vi "REF_EDITOR_records_click_discard.vi"(10 "CellPosition":T2, 11 "event_structure_shift_register_in":T1={"REF_EDIT_clicked_row"=-1, "REF_EDIT_selected_row"=-1, "SQL_EDIT_clicked_row"=-1, "SQL_EDIT_selected_row"=-1, "ARCH_EDIT_selected_row"=-1, "ARCH_EDIT_clicked_row"=-1, "USER_EDIT_selected_row"=-1, "USER_EDIT_clicked_row"=-1, "REPORT_GEAR_toggle_all_results"=FALSE}) -> (2 "Discard?":bool, 3 "event_structure_shift_register_out":T1={"REF_EDIT_clicked_row"=-1, "REF_EDIT_selected_row"=-1, "SQL_EDIT_clicked_row"=-1, "SQL_EDIT_selected_row"=-1, "ARCH_EDIT_selected_row"=-1, "ARCH_EDIT_clicked_row"=-1, "USER_EDIT_selected_row"=-1, "USER_EDIT_clicked_row"=-1, "REPORT_GEAR_toggle_all_results"=FALSE})   [LabVIEW 2019]
uses:
  CLIENT_event_structure_shift_register.ctl
  <vilib>/Utility/miscctls.llb/LVRowAndColumnTypeDef.ctl
  FGV/REF_EDITOR_records_display/FGV_REF_EDITOR_records_display.ctl
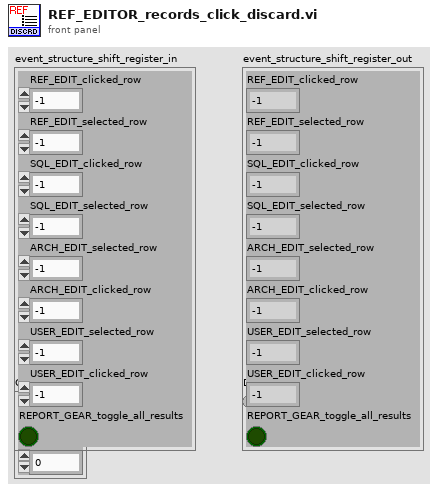
[diagram p1: front panel]
types:
  T1 = typedef "CLIENT_event_structure_shift_register.ctl" = cluster{"REF_EDIT_clicked_row":i32, "REF_EDIT_selected_row":i32, "SQL_EDIT_clicked_row":i32, "SQL_EDIT_selected_row":i32, "ARCH_EDIT_selected_row":i32, "ARCH_EDIT_clicked_row":i32, "USER_EDIT_selected_row":i32, "USER_EDIT_clicked_row":i32, "REPORT_GEAR_toggle_all_results":bool}
  T2 = typedef "LVRowAndColumnTypeDef.ctl" = cluster{"Row":i32, "Column":i32}
  T3 = typedef "FGV_REF_EDITOR_records_display.ctl" = enum16{"initialize", "set_reference_tables_names", "set_station_number", "set_type_filter", "set_headers", "set_records", "get_ref_table_name", "get_ref_hist_table_name", "get_station_number", "get_type_filter", "get_headers", "get_uneditable_columns", "get_all_info", "record_added?", "record_inserted?", "record_edited?", "record_updated?", "record_deleted?", "discard_changes"}
  T4 = typedef "REF_EDITOR_all_info.ctl" = cluster{"station_number":string, "type_filter":string, "reference_table":string, "reference_history":string, "headers":string[], "uneditable_columns":string[], "uneditable_columns":i32[], "editable_columns":i32[], "values_in_database":string[][], "size":cluster{"columns":i32, "SQL_rows":i32, "disp_rows":i32}, "REF_record_states":T5[]}
  T5 = typedef "SQL_record_states.ctl" = enum16{"Equal", "Added", "Edited", "Deleted"}
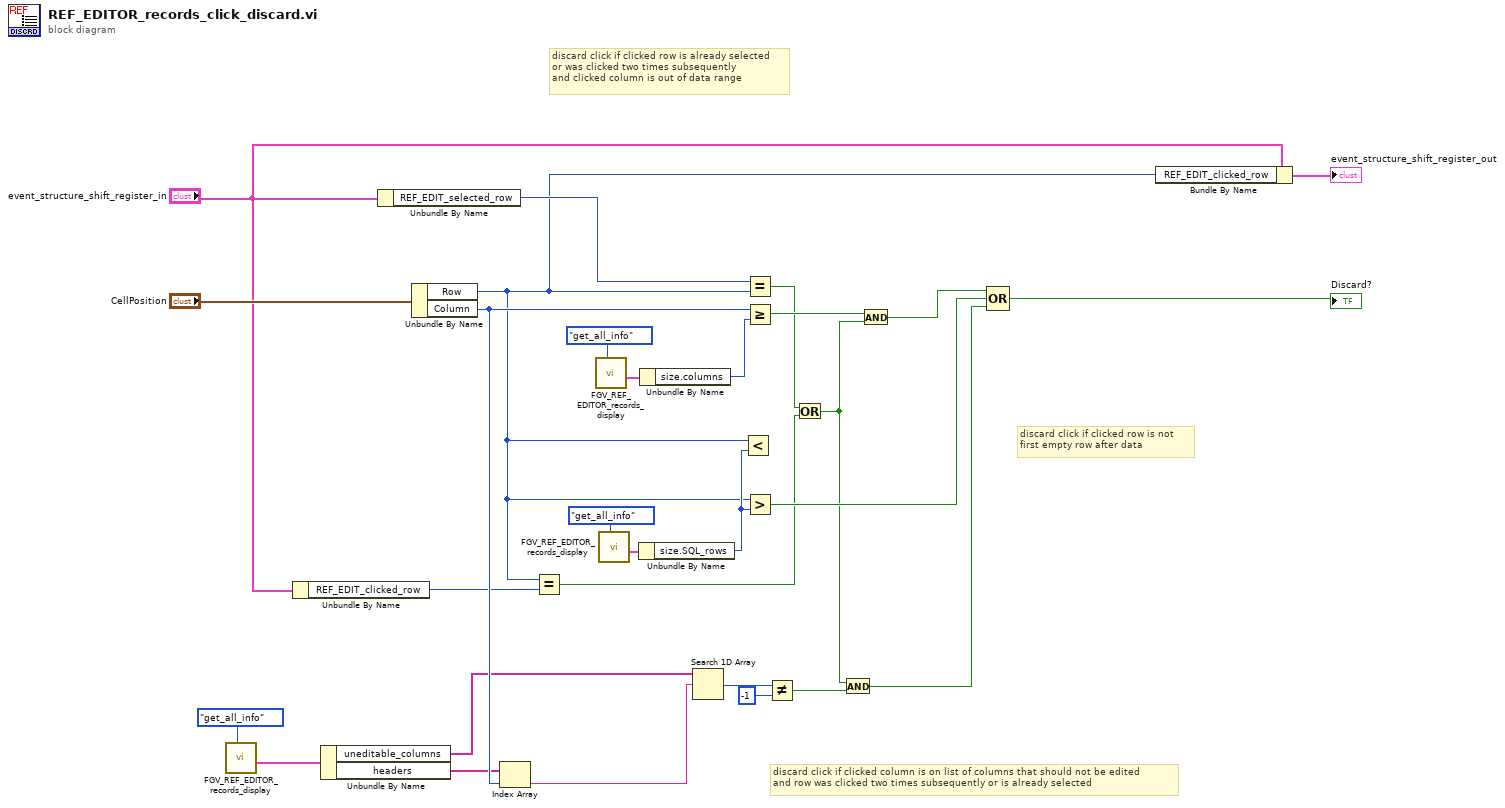
[diagram p0: block diagram]
diagram:
  # "discard click if clicked column is on list of columns that should not be edited\nand row was clicked two times subsequently or is already selected"
  # "discard click if clicked row is not \nfirst empty row after data"
  # "discard click if clicked row is already selected\nor was clicked two times subsequently\nand clicked column is out of data range"
  n1 = call "FGV_REF_EDITOR_records_display.vi"("options"=FGV_REF_EDITOR_records_display."get_all_info") -> ("all_info"=w3:T4)  [unwired: 7 in, 3 out]
  n2 = Unbundle By Name("event_structure_shift_register_in") -> ("REF_EDIT_clicked_row"=w9:i32)
  n3 = Unbundle By Name(w3) -> ("uneditable_columns"=w1:string[], "headers"=w2:string[])
  n4 = Unbundle By Name("event_structure_shift_register_in") -> ("REF_EDIT_selected_row"=w14:i32)
  n5 = Unbundle By Name("CellPosition") -> ("Row"=w8:i32, "Column"=w22:i32)
  n6 = Index Array(array=w2, index=w22) -> (element=w21:string)
  n7 = Equal?(x=w8, y=w9) -> (x = y?=w5:bool)
  n8 = call "FGV_REF_EDITOR_records_display.vi"("options"=FGV_REF_EDITOR_records_display."get_all_info") -> ("all_info"=w26:T4)  [unwired: 7 in, 3 out]
  n9 = call "FGV_REF_EDITOR_records_display.vi"("options"=FGV_REF_EDITOR_records_display."get_all_info") -> ("all_info"=w28:T4)  [unwired: 7 in, 3 out]
  n10 = Unbundle By Name(w28) -> ("size.SQL_rows"=w12:i32)
  n11 = Unbundle By Name(w26) -> ("size.columns"=w25:i32)
  n12 = Search 1D Array(1D array=w1, element=w21) -> (index of element=w20:i32)  [unwired: 1 in]
  n13 = Less?(x=w8, y=w12) -> ()  [unwired: 1 out]
  n14 = Equal?(x=w14, y=w8) -> (x = y?=w6:bool)
  n15 = Greater Or Equal?(x=w22, y=w25) -> (x >= y?=w7:bool)
  n16 = Greater?(x=w8, y=w12) -> (0:w15:bool)
  n17 = Not Equal?(x=w20, y=-1) -> (x != y?=w11:bool)
  n18 = Or(x=w6, y=w5) -> (x .or. y?=w4:bool)
  n19 = And(x=w4, y=w11) -> (x .and. y?=w17:bool)
  n20 = And(x=w7, y=w4) -> (x .and. y?=w18:bool)
  n21 = Compound Arithmetic op=OR(w18, w15, w17) -> (→"Discard?":bool)
  n22 = Bundle By Name(cluster="event_structure_shift_register_in", "REF_EDIT_clicked_row"=w8) -> (→"event_structure_shift_register_out":T1)
